vi "IRHoming2.vi"(9 "Debug?":bool, 10 "Function":u16(ring) items=["Home", "Stop", "Align"], 11 "NXT In":T1) -> (3 "NXT Out":T1)   [LabVIEW 2012]
uses:
  <vilib>/NXT/Subs/LVHSConnector.ctl
  <vilib>/NXT/LegoClasses/BrickReference/BrickReference.lvclass
  <vilib>/NXT/Hardware/Plugins/Tetrix DC Motor/TetrixDCMotorAddress.ctl
  FTC 2012 - 2013/Controls/SpeedControl.ctl
  AutoDriverControl.ctl
  <vilib>/NXT/NXTIO Xnodes/NXTIONodeSubVIs/TETRIX IO Stop DC Motors.vi
  <vilib>/NXT/NXTIO Xnodes/AddressXNode/NXTIOAddress.xnode
  Main/MainProject/MainProject.lvrbt
  <vilib>/NXT/NXTIO Xnodes/NXTIOXNode/NXTIO.xnode
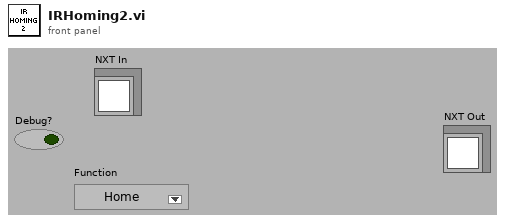
[diagram p1: front panel]
types:
  T1 = typedef "LVHSConnector.ctl" = refnum<class "BrickReference.lvclass">
  T2 = typedef "TetrixDCMotorAddress.ctl" = i16
  T3 = cluster{"TetrixDCMotor":T2, "TetrixDCMotor 2":T2}
  T4 = typedef "AutoDriverControl.ctl" = enum16{"Init", "Forward", "Reverse", "Left", "Right", "Brake"}
  T5 = typedef "SpeedControl.ctl" = enum16{"Fast", "Medium", "Slow"}
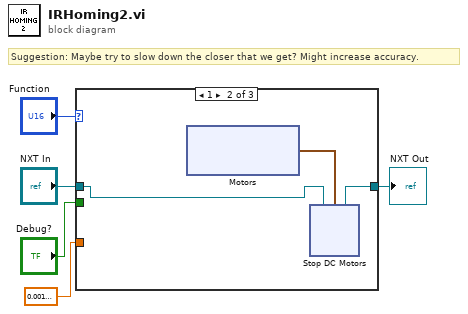
[diagram p0: block diagram]
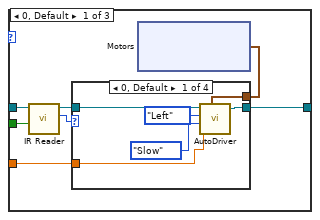
[diagram p2: hidden frame]
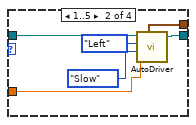
[diagram p3: hidden frame]
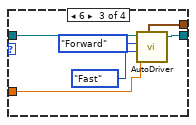
[diagram p4: hidden frame]
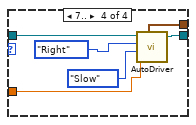
[diagram p5: hidden frame]
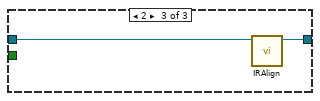
[diagram p6: hidden frame]
diagram:
  # "Suggestion: Maybe try to slow down the closer that we get? Might increase accuracy."
  n1 = case shown="1" "Function" {
    tunnel: "NXT In" -> [w11 w40 w50]
    tunnel: [w12 w39 w49] -> w3
    tunnel: "Debug?" -> [w9 _ _]
    tunnel: sgl 0.001 ("Time (1 sec)") -> [w7 _ _]
    frame 0, Default {
      n2 = call "IR Reader.vi"("Debug"=w9, "NXT In"=w11) -> ("Direction (0-9)"=w8:i16, "NXT Out"=w10:T1)  [unwired: 8 in]
      n3 = xnode "Motors"() -> ("Motor"=w6:cluster{"TetrixDCMotor":T2, "TetrixDCMotor":T2})
      n4 = case shown="0, Default" w8 {
        tunnel: w10 -> [w18 w25 w31 w37]
        tunnel: [w19 w24 w30 w36] -> w12
        tunnel: w7 -> [w16 w22 w28 w34]
        tunnel: w6 -> [w14 w20 w26 w32]
        frame 0, Default {
          n5 = call "AutoDriver.vi"("NXT In"=w18, "Motors"=w14, "Direction"=AutoDriverControl."Left", "Speed"=SpeedControl."Slow", "Time (1 sec)"=w16) -> ("NXT Out"=w19:T1)  [unwired: 3 in]
        }
        frame 1..5 {
          n6 = call "AutoDriver.vi"("NXT In"=w25, "Motors"=w20, "Direction"=AutoDriverControl."Left", "Speed"=SpeedControl."Slow", "Time (1 sec)"=w22) -> ("NXT Out"=w24:T1)  [unwired: 3 in]
        }
        frame 6 {
          n7 = call "AutoDriver.vi"("NXT In"=w31, "Motors"=w26, "Direction"=AutoDriverControl."Forward", "Speed"=SpeedControl."Fast", "Time (1 sec)"=w28) -> ("NXT Out"=w30:T1)  [unwired: 3 in]
        }
        frame 7.. {
          n8 = call "AutoDriver.vi"("NXT In"=w37, "Motors"=w32, "Direction"=AutoDriverControl."Right", "Speed"=SpeedControl."Slow", "Time (1 sec)"=w34) -> ("NXT Out"=w36:T1)  [unwired: 3 in]
        }
      }
    }
    frame 1 {
      n9 = xnode "Motors"() -> ("Motor"=w38:cluster{"TetrixDCMotor":T2, "TetrixDCMotor":T2})
      n10 = xnode "Stop DC Motors"("Motors"=w38, "NXT"=w40) -> ("NXT"=w39:T1)
    }
    frame 2 {
      n11 = call "IRAlign.vi"("NXT"=w50) -> ("NXT Out"=w49:T1)  [unwired: 10 in]
    }
  }
  "NXT Out" <- w3
